vi "save.volume.vi"(7 "id":i32, 8 "error in (no error)":errorcluster, 11 "volume":T1) -> (0 "error out":errorcluster, 3 "volume out":T1)   [LabVIEW 2024, in "manager_daemon.lvclass"]
uses:
  manager_daemon.lvclass
  manager_daemon.lvclass/manager_daemon.ctl
  CV_Shared_Library/volume.type--enum.ctl
  CV_Shared_Library/CV_Shared_Library.lvlib
  CV_RESTful_Library/typedefs/local_volume--cluster.ctl
  CV_RESTful_Library/CV_RESTful_Lib.lvlib
  <vilib>/addons/_JKI.lib/Serialization/JSON/JKI JSON Serialization.lvlib
  type_defs/VolumeData--cluster.ctl
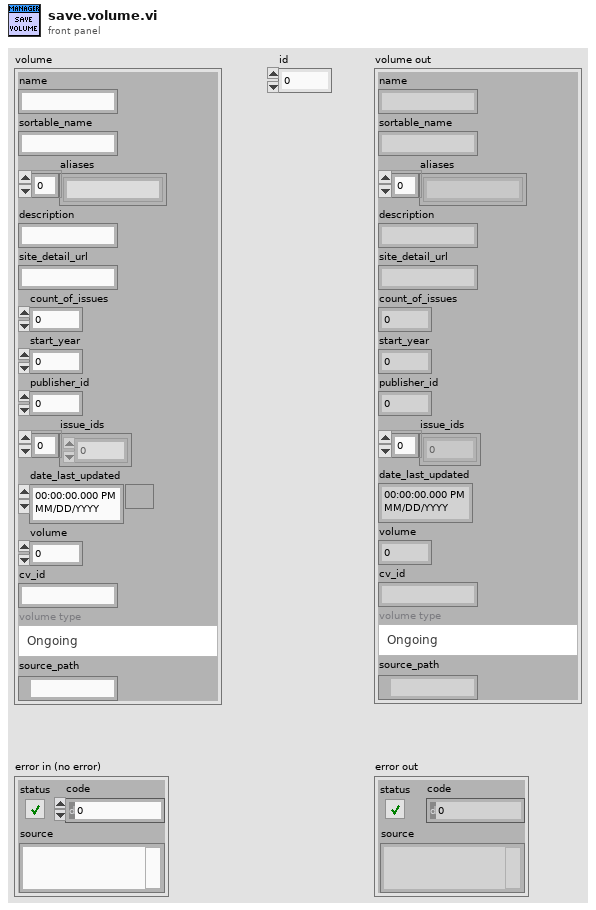
[diagram p1: front panel]
types:
  T1 = typedef "manager_daemon.lvclass/VolumeData--cluster.ctl" = cluster{"name":string, "sortable_name":string, "aliases":string[], "description":string, "site_detail_url":string, "count_of_issues":i32, "start_year":i32, "publisher_id":i32, "issue_ids":i32[], "date_last_updated":timestamp, "volume":i32, "cv_id":string, "volume type":T2, "source_path":path}
  T2 = typedef "CV_Shared_Library.lvlib/volume.type--enum.ctl" = enum16{"Ongoing", "Limited Series", "Annual", "One Shot", "Reprint/Document", "Star Comics", "Epic Comics"}
  T3 = typedef "CV_RESTful_Lib.lvlib/local_volume--cluster.ctl" = cluster{"id":i32, "name":string, "sortable_name":string, "aliases":string[], "description":string, "site_detail_url":string, "count_of_issues":i32, "start_year":i32, "publisher_id":i32, "issue_ids":i32[], "date_last_updated":timestamp, "volume":i32, "cv_id":string, "volume type":T2}
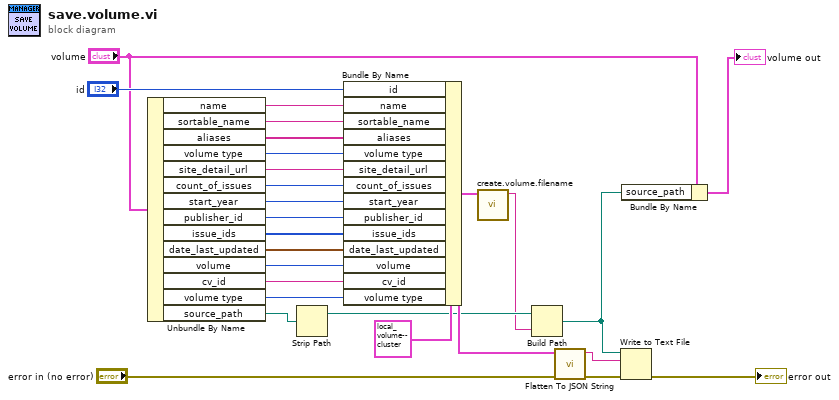
[diagram p0: block diagram]
diagram:
  n1 = Unbundle By Name("volume") -> ("name"=w25:string, "sortable_name"=w23:string, "aliases"=w22:string[], "volume type"=w21:T2, "site_detail_url"=w20:string, "count_of_issues"=w19:i32, "start_year"=w18:i32, "publisher_id"=w17:i32, "issue_ids"=w16:i32[], "date_last_updated"=w15:timestamp, "volume"=w14:i32, "cv_id"=w13:string, "volume type"=w12:T2, "source_path"=w6:path)
  n2 = Strip Path(path=w6) -> (stripped path=w5:path)  [unwired: 1 out]
  n3 = Bundle By Name(cluster=T3 {"id"=0, "name"="", "sortable_name"="", "aliases"=[], "description"="", "site_detail_url"="", "count_of_issues"=0, "start_year"=0, "publisher_id"=0, "issue_ids"=[], "date_last_updated"=timestamp(0 s since 1904-01-01), "volume"=0, "cv_id"="", "volume type"=enum."One Shot"} ("local volume"), "id"="id", "name"=w25, "sortable_name"=w23, "aliases"=w22, "volume type"=w21, "site_detail_url"=w20, "count_of_issues"=w19, "start_year"=w18, "publisher_id"=w17, "issue_ids"=w16, "date_last_updated"=w15, "volume"=w14, "cv_id"=w13, "volume type"=w12) -> (w7:T3)
  n4 = call "create.volume.filename.vi"("volume"=w7) -> ("json filename"=w4:string)  [unwired: 10 in]
  n5 = Build Path(base path=w5, name or relative path=w4) -> (appended path=w2:path)
  n6 = call <vilib>:"Flatten To JSON String.vi"("error in"="error in (no error)", "Variant"=w7) -> ("error out"=w10:errorcluster, "JSON String"=w8:string)  [unwired: 8 in]
  n7 = Write to Text File(file (use dialog)=w2, text=w8, error in=w10) -> (error out=→"error out":errorcluster)  [unwired: 1 in, 2 out]
  n8 = Bundle By Name(cluster="volume", "source_path"=w2) -> (→"volume out":T1)
